vi "Export_FreDomain_Data.vi"(0 "nCmdShow":i16(ring) items=["SW_HIDE   ", "SW_SHOWNORMAL", "SW_SHOWMINIMIZED", "SW_SHOWMAXIMIZED", "SW_SHOWNOACTIVATE", "SW_SHOW", "SW_MINIMIZE", "SW_SHOWMINNOACTIVE", "SW_SHOWNA", "SW_RESTORE"], 2 "szFileName":string="D:\\TX1.s4p", 4 "delimiterType":i16(ring) items=["Tab", "Comma"], 6 "Port Type":u16(ring)) -> (20 "Single S-parameters Data":dbl[][](array[numeric]), 22 "Diff S-parameters Data":dbl[][](array[numeric]), 24 "Frequency":dbl[](array[numeric]), 27 "S-parameter Chart":cluster{dbl[], "Diff S-parameters Data":dbl[]}[](graph))   [LabVIEW 2011]
uses:
  Data/Interop.PLTS.dll
  <vilib>/Utility/file.llb/Read From Spreadsheet File (string).vi
  <vilib>/Utility/file.llb/Read From Spreadsheet File (DBL).vi
panel:
  in  "StepFreqMHz":dbl=10.0
  in  "StartFreqMHz":dbl=10.0
  in  "Freq Unit":i16(ring) items=["MHz", "GHz"]
  in  "AnalysisType":i16(ring)=2 items=["TIME_DIFF  ", "TIME_SNGL", "FREQ_BAL", "FREQ_SNGL"]
  in  "dataFormat":i16(ring) items=["RI", "LogMag", "Linear", "Phase"]
  in  "ParamList":string="SDD11"
  in  "StopFreqMHz":dbl=10000.0
  in  "dataToExport":i16(ring) items=["SE", "Balanced", "All ", "Customized"]
  in  "FileName":string="D:\\111.txt"
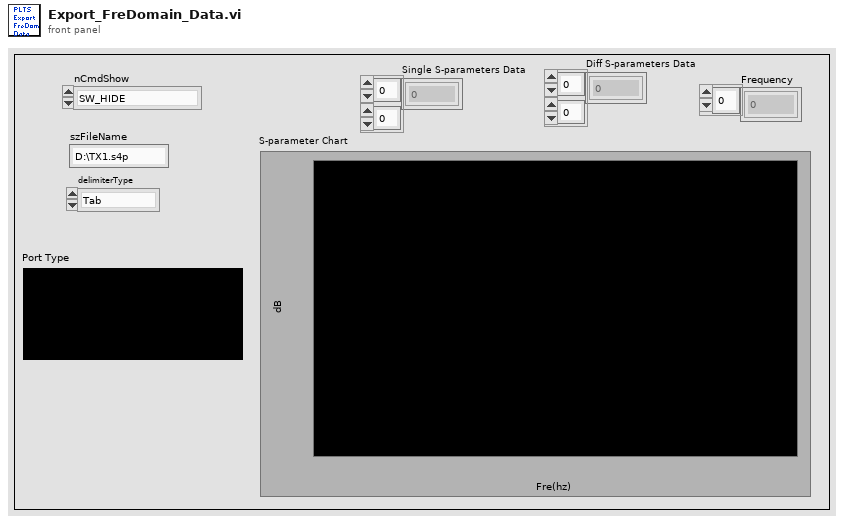
[diagram p1: front panel]
types:
  T1 = enum16{"SDD21", "SDD12", "SDD11", "SDD22", "SCD21", "SCD12", "SCD22", "SCD11", "SDC11", "SDC22", "SDC12", "SDC21", "SCC11", "SCC22", "SCC12", "SCC21"}
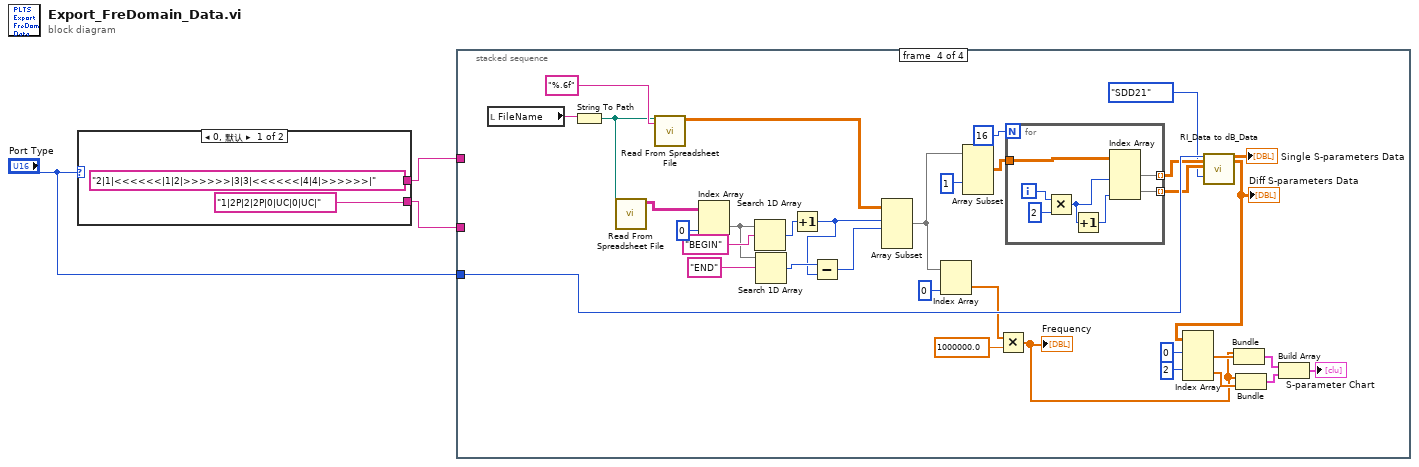
[diagram p0: block diagram]
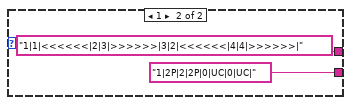
[diagram p2: hidden frame]
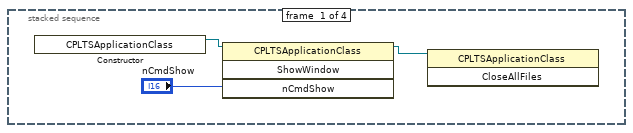
[diagram p3: hidden frame]
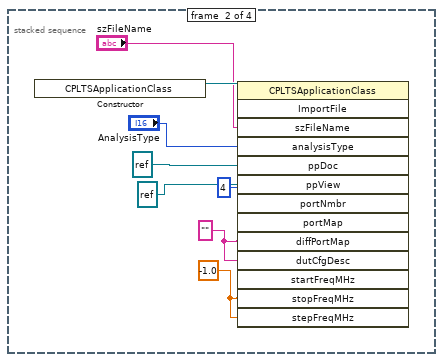
[diagram p4: hidden frame]
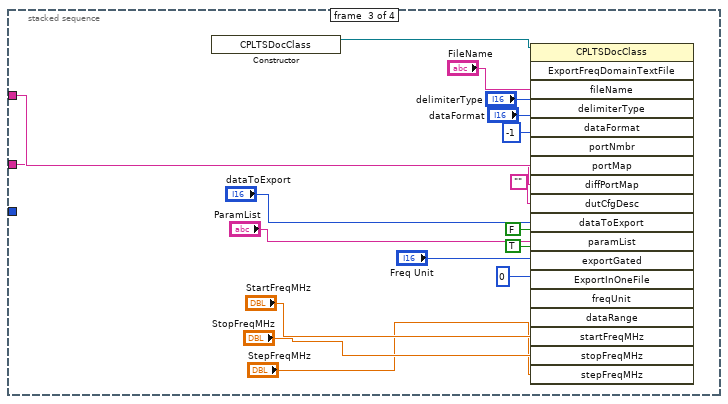
[diagram p5: hidden frame]
diagram:
  n1 = case shown="0, 默认" "Port Type" {
    tunnel: ["2|1|<<<<<<|1|2|>>>>>>|3|3|<<<<<<|4|4|>>>>>>|" ("portMap") "1|1|<<<<<<|2|3|>>>>>>|3|2|<<<<<<|4|4|>>>>>>|" ("portMap")] -> w3
    tunnel: ["1|2P|2|2P|0|UC|0|UC|" ("diffPortMap") "1|2P|2|2P|0|UC|0|UC|" ("diffPortMap")] -> w2
    frame 0, Default {
    }
    frame 1 {
    }
  }
  n2 = stacked-sequence {
    tunnel: w3 -> [_ _ w30 _]
    tunnel: w2 -> [_ _ w29 _]
    tunnel: "Port Type" -> [_ _ _ w51]
    frame #0 {
      n3 = constructor class="CPLTSApplicationClass"() -> (reference out=w10:refnum<k24>)  [unwired: 3 in, 2 out]
      n4 = invoke class="CPLTSApplicationClass" method="ShowWindow"(reference=w10, "nCmdShow"="nCmdShow") -> (reference out=w8:refnum<k24>)  [unwired: 2 in, 3 out]
      n5 = invoke class="CPLTSApplicationClass" method="CloseAllFiles"(reference=w8) -> ()  [unwired: 2 in, 3 out]
    }
    frame #1 {
      w12 = -1.0 ("startFreqMHz")
      w14 = "" ("portMap")
      n6 = constructor class="CPLTSApplicationClass"() -> (reference out=w18:refnum<k24>)  [unwired: 3 in, 2 out]
      n7 = invoke class="CPLTSApplicationClass" method="ImportFile"(reference=w18, "szFileName"="szFileName", "analysisType"="AnalysisType", "ppDoc"=refnum<k24> refnum, "ppView"=refnum<k24> refnum, "portNmbr"=i16 4, "portMap"=w14, "diffPortMap"=w14, "dutCfgDesc"=w14, "startFreqMHz"=w12, "stopFreqMHz"=w12, "stepFreqMHz"=w12) -> ()  [unwired: 2 in, 14 out]
    }
    frame #2 {
      n8 = constructor class="CPLTSDocClass"() -> (reference out=w35:refnum<k24>)  [unwired: 3 in, 2 out]
      n9 = invoke class="CPLTSDocClass" method="ExportFreqDomainTextFile"(reference=w35, "fileName"="FileName", "delimiterType"="delimiterType", "dataFormat"="dataFormat", "portNmbr"=i16 -1, "portMap"=w30, "diffPortMap"=w29, "dutCfgDesc"="", "dataToExport"="dataToExport", "paramList"="ParamList", "exportGated"=FALSE ("ExportInOneFile"), "ExportInOneFile"=TRUE, "freqUnit"="Freq Unit", "dataRange"=i16 0, "startFreqMHz"="StartFreqMHz", "stopFreqMHz"="StopFreqMHz", "stepFreqMHz"="StepFreqMHz") -> ()  [unwired: 2 in, 19 out]
    }
    frame #3 {
      n10 = local read "FileName"() -> (w69:string)
      n11 = String To Path(string=w69) -> (path=w65:path)
      n12 = call-poly <vilib>:"Read From Spreadsheet File.vi"("file path (dialog if empty)"=w65) -> ("all rows"=w64:string[][])  [unwired: 6 in, 4 out]
      n13 = call-poly <vilib>:"Read From Spreadsheet File.vi"("format (%.3f)"="%.6f", "file path (dialog if empty)"=w65) -> ("all rows"=w67:dbl[][])  [unwired: 5 in, 4 out]
      n14 = Index Array(array=w64, index (col)=0 ("禁用的索引 (列)")) -> (element=w62:string[])  [unwired: 1 in]
      n15 = Search 1D Array(1D array=w62, element="BEGIN" ("元素")) -> (index of element=w59:i32)  [unwired: 1 in]
      n16 = Search 1D Array(1D array=w62, element="END" ("元素")) -> (index of element=w60:i32)  [unwired: 1 in]
      n17 = Increment(x=w59) -> (x+1=w57:i32)
      n18 = Subtract(x=w60, y=w57) -> (x-y=w58:i32)
      n19 = Array Subset(array=w67, index (row)=w57, length (row)=w58) -> (w52:dbl[][])  [unwired: 2 in]
      n20 = Index Array(array=w52, index (col)=0 ("禁用的索引 (列)")) -> (element=w37:dbl[])  [unwired: 1 in]
      n21 = Array Subset(array=w52, index (col)=1 ("索引")) -> (w54:dbl[][])  [unwired: 3 in]
      n22 = Multiply(x=w37, y=1000000.0) -> (x*y=w36:dbl[])
      "Frequency" <- w36
      n23 = for {
        N: 16 -> [_]
        tunnel: w54 -> [w76]
        tunnel: [w71] -> w50 mode=indexing
        tunnel: [w70] -> w49 mode=indexing
        i -> [w75]
        n24 = Multiply(x=w75, y=2) -> (x*y=w73:i32)
        n25 = Increment(x=w73) -> (x+1=w72:i32)
        n26 = Index Array(array=w76, index (col) #1=w73, index (col) #2=w72) -> (element #1=w71:dbl[], element #2=w70:dbl[])  [unwired: 2 in]
      }
      n27 = call "RI_Data to dB_Data.vi"("Port Type"=w51, "Sxx_R"=w50, "Sxx_I"=w49, "S-Parameter Name"=T1."SDD21") -> ("Single S-parameters Data"=→"Single S-parameters Data":dbl[][], "Diff S-parameters Data"=w47:dbl[][])  [unwired: 14 in]
      "Diff S-parameters Data" <- w47
      n28 = Index Array(array=w47, index (row) #1=0 ("索引 (行)"), index (row) #2=2 ("索引 (行)")) -> (element #1=w45:dbl[], element #2=w43:dbl[])  [unwired: 2 in]
      n29 = Bundle(w36, "Diff S-parameters Data"=w45) -> (w42:cluster{dbl[], "Diff S-parameters Data":dbl[]})  [unwired: 1 in]
      n30 = Bundle(w36, "Diff S-parameters Data"=w43) -> (w41:cluster{dbl[], "Diff S-parameters Data":dbl[]})  [unwired: 1 in]
      n31 = Build Array(w42, w41) -> (→"S-parameter Chart":cluster{dbl[], "Diff S-parameters Data":dbl[]}[])
    }
  }
